vi "decimate-points_multiple_axis.vi"(7 "type":T1, 8 "error in (no error)":errorcluster, 9 "height_width":u32, 10 "y_axis in":dbl[][](array[numeric]), 11 "x_axis in":dbl[](array[numeric])) -> (0 "error out":errorcluster, 2 "y_axis out":dbl[][](array[numeric]), 3 "x_axis out":dbl[](array[numeric]))   [LabVIEW 2015, in "lv-graph.lvlib"]
doc: "This VI will decimate a given dataset, following the rule that you can display, at most two points per pixel per plot. If the number of points exceeds the number of pixels (wired from height_width). For decimation, it'll group equal sets of points (except the last set) for data representation. As configured, the way the points are represented can be configured as follows: (1) average: this will get the mean of the points per group (2) min_max will average the min/max values for the group (3) max: will return the max value, (4) min: will return the min value, (5) first will return the first value and (6) last will return the last value."
uses:
  lv-graph.lvlib
  _controls/decimation_type.ctl
  <vilib>/Analysis/baseanly.llb/Mean (DBL).vi
  <vilib>/Analysis/NI_AALBase.lvlib
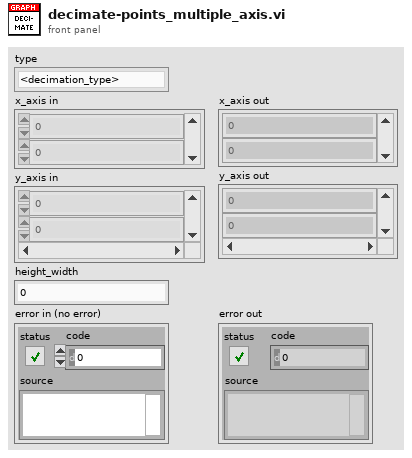
[diagram p1: front panel]
types:
  T1 = typedef "lv-graph.lvlib/decimation_type.ctl" = enum16{"<decimation_type>", "average", "min_max", "max", "min", "first", "last"}
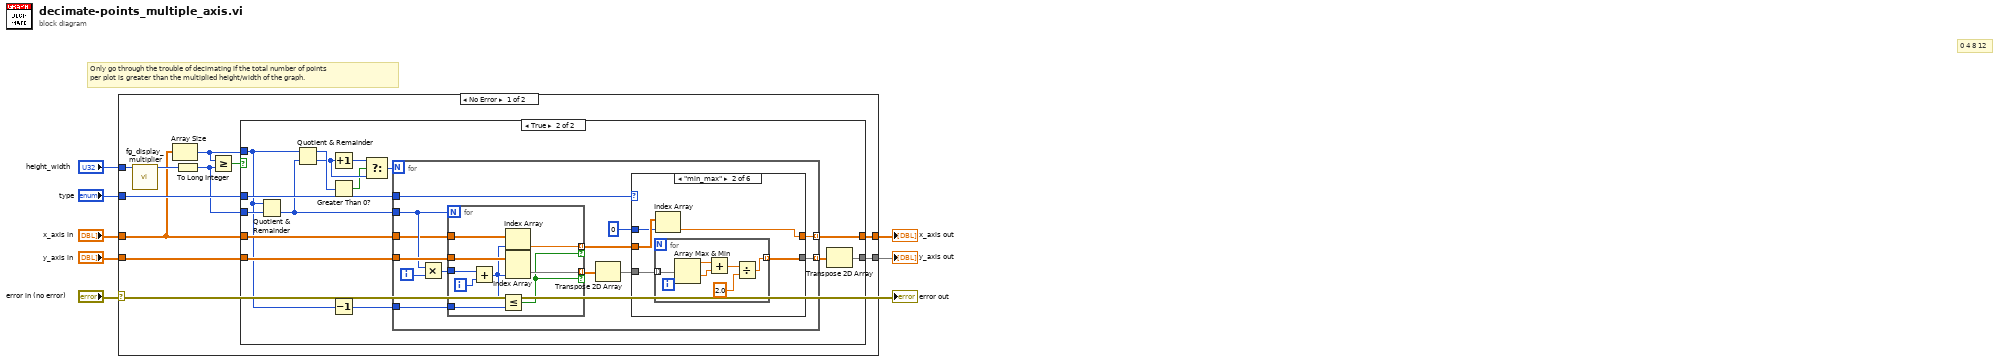
[diagram p0: block diagram]
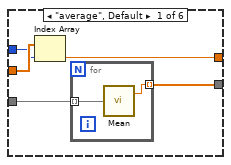
[diagram p3: hidden frame]
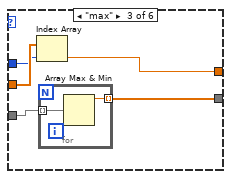
[diagram p4: hidden frame]
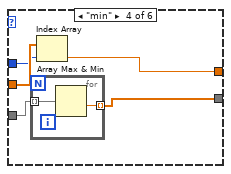
[diagram p5: hidden frame]
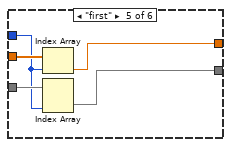
[diagram p6: hidden frame]
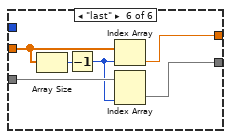
[diagram p7: hidden frame]
diagram:
  # "Only go through the trouble of decimating if the total number of points\nper plot is greater than the multiplied height/width of the graph."
  # "0 4 8 12"
  n1 = case shown="No Error" "error in (no error)" {
    tunnel: "height_width" -> [w17 _]
    tunnel: "x_axis in" -> [w8 _]
    tunnel: "y_axis in" -> [w16 _]
    tunnel: "type" -> [w15 _]
    tunnel: [w14 _] -> w3
    tunnel: [w13 _] -> w2
    frame No Error {
      n2 = call "fg_display_multiplier.vi"("width_height in"=w17) -> ("width_height out"=w10:u32)  [unwired: 9 in, 1 out]
      n3 = Array Size(array=w8) -> (size(s)=w12:i32)
      n4 = To Long Integer(number=w10) -> (32bit integer=w9:i32)
      n5 = Greater Or Equal?(x=w12, y=w9) -> (x >= y?=w11:bool)
      n6 = case shown="True" w11 {
        tunnel: w8 -> [w19 w30]
        tunnel: w16 -> [w18 w29]
        tunnel: w15 -> [_ w28]
        tunnel: w12 -> [_ w23]
        tunnel: w9 -> [_ w27]
        tunnel: [w19 w26] -> w14
        tunnel: [w18 w20] -> w13
        frame False {
        }
        frame True {
          n7 = Quotient & Remainder(x=w23, y=w27) -> (floor(x/y)=w24:i32)  [unwired: 1 out]
          n8 = Quotient & Remainder(x=w23, y=w24) -> (x-y*floor(x/y)=w34:i32, floor(x/y)=w33:i32)
          n9 = Increment(x=w33) -> (x+1=w31:i32)
          n10 = Greater Than 0?(x=w34) -> (x > 0?=w25:bool)
          n11 = Decrement(x=w23) -> (x-1=w22:i32)
          n12 = Select(t=w31, s=w25, f=w33) -> (s? t:f=w32:i32)
          n13 = for {
            N: w32 -> [_]
            tunnel: w24 -> [w41]
            tunnel: w30 -> [w38]
            tunnel: w29 -> [w47]
            tunnel: w28 -> [w45]
            tunnel: [w43] -> w21 mode=indexing
            tunnel: [w42] -> w26 mode=indexing
            tunnel: w22 -> [w37]
            i -> [w46]
            n14 = Multiply(x=w41, y=w46) -> (x*y=w40:i32)
            n15 = for {
              N: w41 -> [_]
              tunnel: w38 -> [w99]
              tunnel: w47 -> [w98]
              tunnel: w40 -> [w95]
              tunnel: [w97] -> w44 mode=indexing if=w92
              tunnel: [w96] -> w36 mode=indexing if=w92
              tunnel: w37 -> [w93]
              i -> [w94]
              n16 = Add(x=w95, y=w94) -> (x+y=w91:i32)
              n17 = Less Or Equal?(x=w91, y=w93) -> (x <= y?=w92:bool)
              n18 = Index Array(array=w99, index=w91) -> (element=w97:dbl)
              n19 = Index Array(array=w98, index (col)=w91) -> (element=w96:dbl[])  [unwired: 1 in]
            }
            n20 = Transpose 2D Array(2D array=w36) -> (transposed array=w35:dbl[][])
            n21 = case shown="\"min_max\"" w45 {
              tunnel: w44 -> [w49 w57 w68 w75 w84 w88]
              tunnel: w35 -> [w52 w59 w70 w77 w83 w86]
              tunnel: [w51 w58 w69 w76 w80 w89] -> w43
              tunnel: [w50 w56 w67 w74 w81 w90] -> w42
              tunnel: 0 ("index") -> [w48 w55 w66 w73 w82 _]
              frame "average", Default {
                n22 = Index Array(array=w49, index=w48) -> (element=w50:dbl)
                n23 = for {
                  tunnel: w52 -> [w54] mode=indexing
                  tunnel: [w53] -> w51 mode=indexing
                  n24 = call-poly <vilib>:"Mean.vi"("X"=w54) -> ("mean"=w53:dbl)  [unwired: 1 out]
                }
              }
              frame "min_max" {
                n25 = for {
                  tunnel: w59 -> [w65] mode=indexing
                  tunnel: [w60] -> w58 mode=indexing
                  n26 = Array Max & Min(array=w65) -> (max value=w64:dbl, min value=w63:dbl)  [unwired: 2 out]
                  n27 = Add(x=w64, y=w63) -> (x+y=w62:dbl)
                  n28 = Divide(x=w62, y=2.0) -> (x/y=w60:dbl)
                }
                n29 = Index Array(array=w57, index=w55) -> (element=w56:dbl)
              }
              frame "max" {
                n30 = Index Array(array=w68, index=w66) -> (element=w67:dbl)
                n31 = for {
                  tunnel: w70 -> [w72] mode=indexing
                  tunnel: [w71] -> w69 mode=indexing
                  n32 = Array Max & Min(array=w72) -> (max value=w71:dbl)  [unwired: 3 out]
                }
              }
              frame "min" {
                n33 = for {
                  tunnel: w77 -> [w79] mode=indexing
                  tunnel: [w78] -> w76 mode=indexing
                  n34 = Array Max & Min(array=w79) -> (min value=w78:dbl)  [unwired: 3 out]
                }
                n35 = Index Array(array=w75, index=w73) -> (element=w74:dbl)
              }
              frame "first" {
                n36 = Index Array(array=w84, index=w82) -> (element=w81:dbl)
                n37 = Index Array(array=w83, index (col)=w82) -> (element=w80:dbl[])  [unwired: 1 in]
              }
              frame "last" {
                n38 = Array Size(array=w88) -> (size(s)=w87:i32)
                n39 = Decrement(x=w87) -> (x-1=w85:i32)
                n40 = Index Array(array=w88, index=w85) -> (element=w90:dbl)
                n41 = Index Array(array=w86, index (col)=w85) -> (element=w89:dbl[])  [unwired: 1 in]
              }
            }
          }
          n42 = Transpose 2D Array(2D array=w21) -> (transposed array=w20:dbl[][])
        }
      }
    }
    frame Error {
    }
  }
  "x_axis out" <- w3
  "y_axis out" <- w2
  "error out" <- "error in (no error)"
